vi "Test Event Manager API.vi"() -> ()   [LabVIEW 2022 SP3]
doc: "Event Manager API Tester.\n\n<b>Note:</b> This VI was modified by the <b>Validate DQMH Module</b> tool to add the 'Show Main VI Diagram on Init' functionality included in DQMH 6.1.\n\n<b>Note:</b> This VI was modified by the <b>Validate DQMH Module</b> tool to upgrade its Error Reported event frame to use an improved mechanism for displaying error information.\n\n____\nHAMPEL SOFTWARE ENGINEERING v2.6.0 (2023-12-19 10:54)"
uses:
  Libraries/hse-libraries/Source/hse-dqmh/Controls/Module Display Scenarios.ctl
  <vilib>/Utility/error.llb/DialogType.ctl
  <vilib>/Hampel Software Engineering/HSE Logger/LogRecord/LogRecord.lvclass/LogRecord.ctl
  Event Manager.lvlib
  <vilib>/Hampel Software Engineering/HSE Logger/hse-logger.lvlib
  Libraries/hse-libraries/Source/hse-dqmh/hse-dqmh.lvlib
  <vilib>/Hampel Software Engineering/HSE Logger/LogRecord/LogRecord.lvclass
panel:
  in  "Show Main VI Diagram on Init (F)":bool
  in  "Request UI Display":bool
  in  "Prepare":bool
  in  "Configure":bool
  in  "Scenario":T1
  in  "Set Modules":bool
  in  "Module Paths":path[](array[path])=[path "Modules/Dummie"]
  in  "btn_CRITICAL":bool
  in  "btn_ERROR":bool
  in  "btn_WARNING":bool
  in  "btn_INFO":bool
  in  "btn_DEBUG":bool
  in  "Message":string
  in  "Log Error":errorcluster
  out "Log Record":T2
  in  "Show Block Diagram":bool
  in  "Stop Module":bool
  in  "Start Module":bool
  in  "Hide Module Panel":bool
  in  "Show Module Panel":bool
  out "Status":string
  out "Module Running?":bool
  # "CRITICAL Event"
  # "Generate Event"
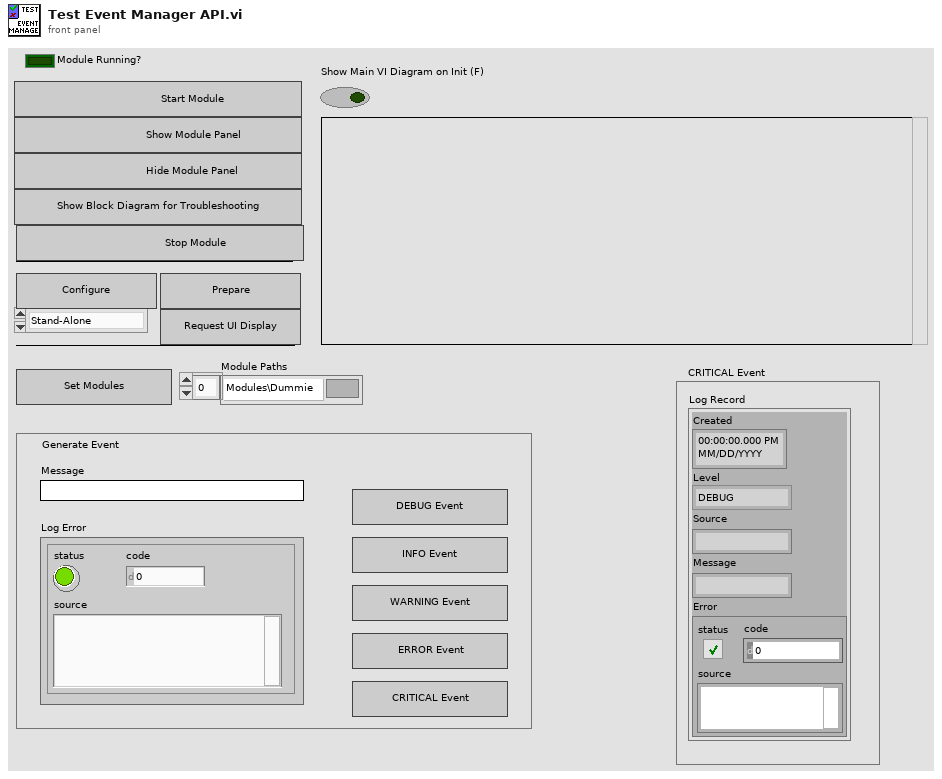
[diagram p1: front panel]
types:
  T1 = typedef "hse-dqmh.lvlib/Module Display Scenarios.ctl" = enum16{"Stand-Alone", "Managed"}
  T2 = cluster{"Created":timestamp, "Level":enum16{"DEBUG", "INFO", "WARNING", "ERROR", "CRITICAL"}, "Source":string, "Message":string, "Error":errorcluster}
  T3 = typedef "Event Manager.lvlib/Broadcast Events--cluster.ctl" = cluster{"Module Did Init":refnum<user-event>, "Status Updated":refnum<user-event>, "Error Reported":refnum<user-event>, "Module Did Stop":refnum<user-event>, "Update Module Execution Status":refnum<user-event>, "System Message":refnum<user-event>}
  T4 = typedef "DialogType.ctl" = u16
  T5 = typedef "hse-dqmh.lvlib/System Message Source.ctl" = enum16{"module", "application", "network"}
  T6 = typedef "hse-logger.lvlib/LogLevel.ctl" = enum16{"DEBUG", "INFO", "WARNING", "ERROR", "CRITICAL"}
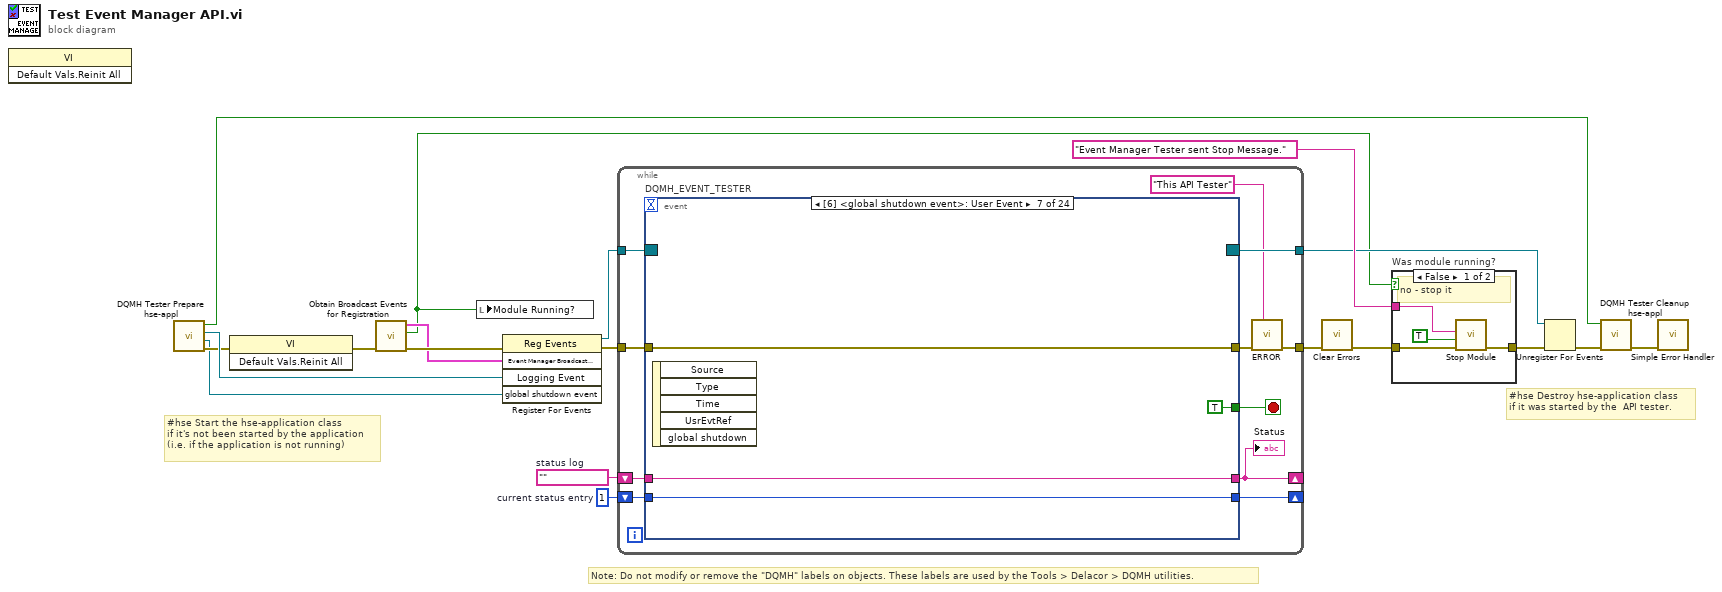
[diagram p0: block diagram]
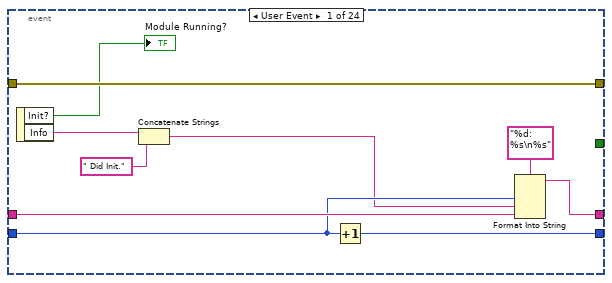
[diagram p3: hidden frame]
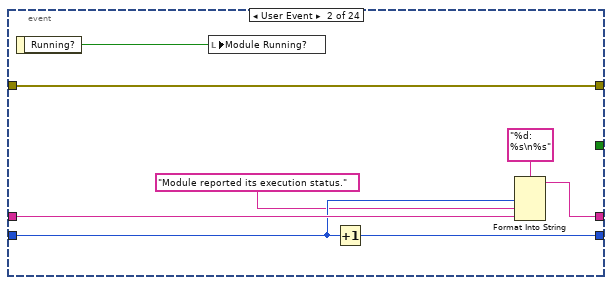
[diagram p4: hidden frame]
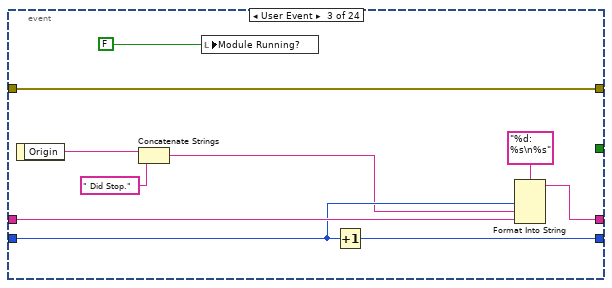
[diagram p5: hidden frame]
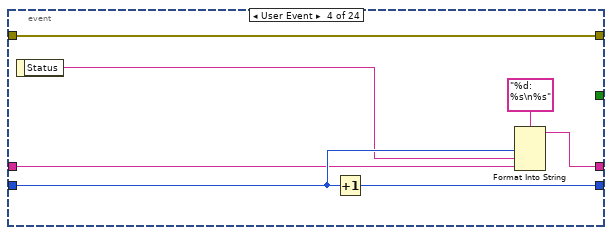
[diagram p6: hidden frame]
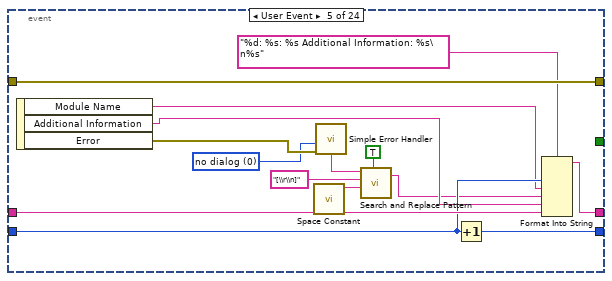
[diagram p7: hidden frame]
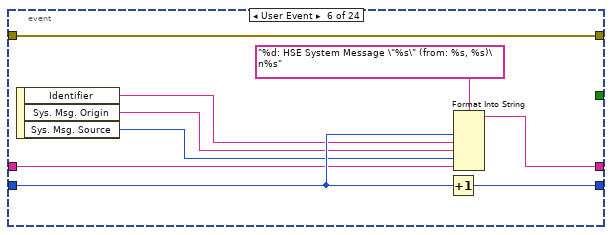
[diagram p8: hidden frame]
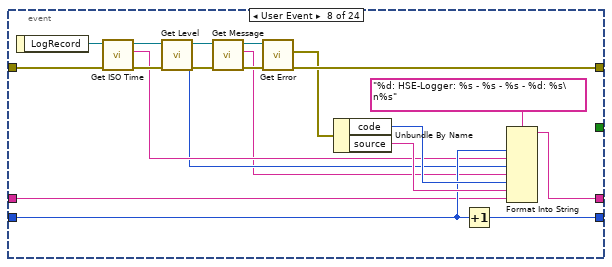
[diagram p9: hidden frame]
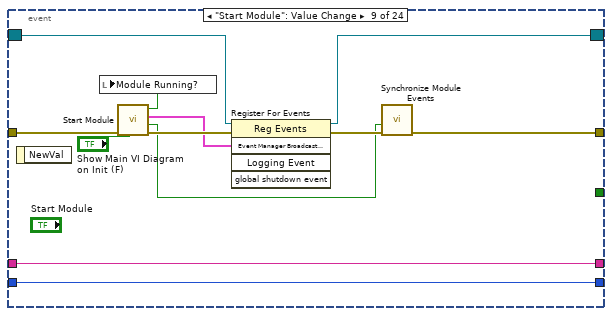
[diagram p10: hidden frame]
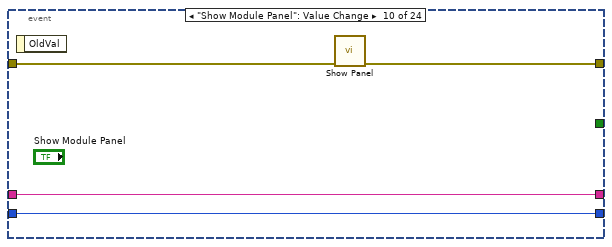
[diagram p11: hidden frame]
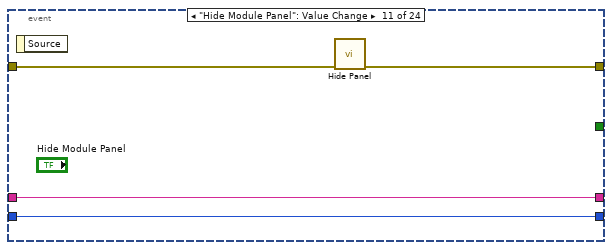
[diagram p12: hidden frame]
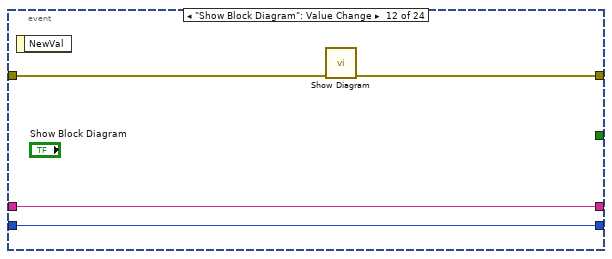
[diagram p13: hidden frame]
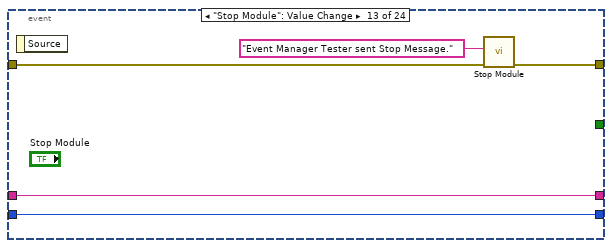
[diagram p14: hidden frame]
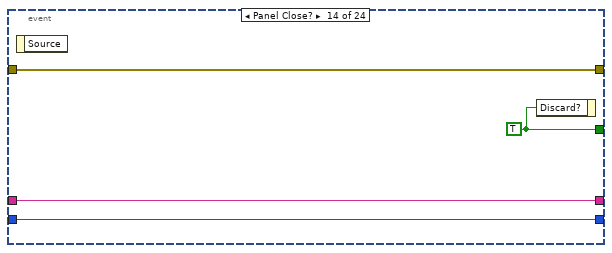
[diagram p15: hidden frame]
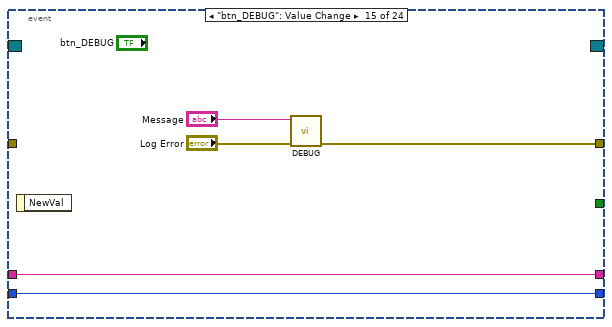
[diagram p16: hidden frame]
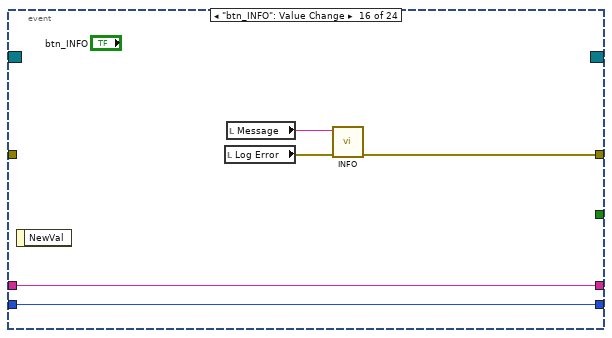
[diagram p17: hidden frame]
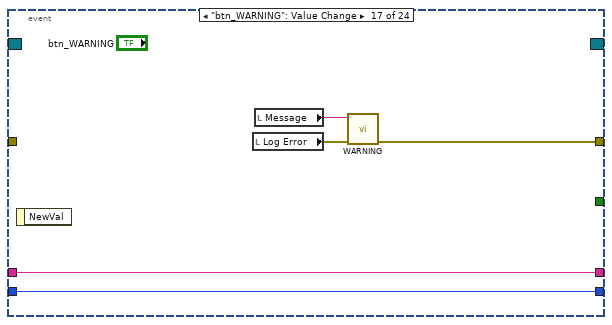
[diagram p18: hidden frame]
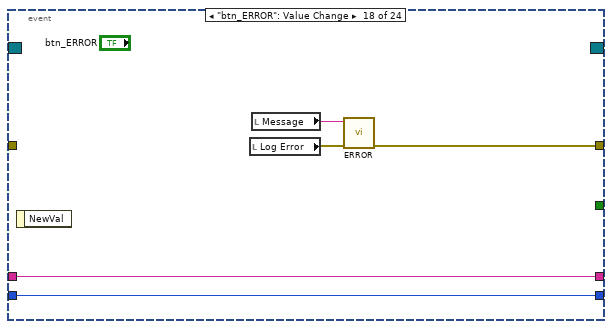
[diagram p19: hidden frame]
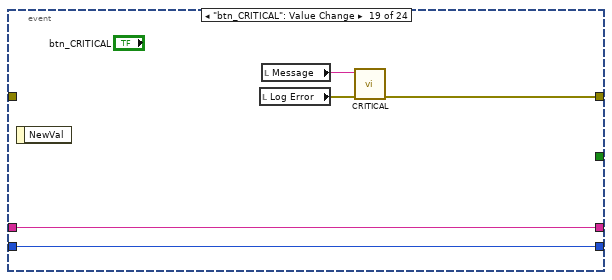
[diagram p20: hidden frame]
diagram:
  w17 = 1  # current status entry
  w18 = ""  # status log
  # "#hse Destroy hse-application class \nif it was started by the  API tester."
  # "#hse Start the hse-application class \nif it's not been started by the application\n(i.e. if the application is not running)"
  # "Note: Do not modify or remove the \"DQMH\" labels on objects. These labels are used by the Tools > Delacor > DQMH utilities."
  n1 = invoke class="VI" method="Default Vals.Reinit All"() -> ()  [unwired: 3 in, 3 out]
  n2 = call "DQMH Tester Prepare hse-appl.vi"() -> ("error out"=w9:errorcluster, "global shutdown event"=w1:refnum<user-event>, "Logging Event"=w10:refnum<user-event>, "Started?"=w12:bool)  [unwired: 8 in]
  n3 = invoke class="VI" method="Default Vals.Reinit All"(error in=w9) -> (error out=w8:errorcluster)  [unwired: 2 in, 2 out]
  n4 = call "Obtain Broadcast Events for Registration.vi"("error in (no error)"=w8) -> ("error out"=w7:errorcluster, "Already running?"=w3:bool, "Event Manager Broadcast Events"=w6:T3)  [unwired: 8 in]
  n5 = local write "Module Running?"(w3) -> ()
  n6 = register-events(error in=w7, w6, w10, w1) -> (reference out=w15:refnum<event-registration>, error out=w16:errorcluster)  [unwired: 1 in]
  n7 = while {
    tunnel: w15 -> [w30]
    tunnel: [w21] -> w13
    shift-right: [w26] -> _
    shift-left: w18 -> [w28]
    shift-right: [w27] -> _
    shift-left: w17 -> [w29]
    tunnel: w16 -> [w25]
    tunnel: [w24] -> w14
    stop <- w22 stop-if-true
    n8 = event "DQMH_EVENT_TESTER" shown="[6] <global shutdown event>: User Event" {
      selector: w30 -> [_ _ _ _ _ _ _ _ w119 _ _ _ _ _ _ _ _ _ _ _ _ _ _ _]
      dyn-events: [_ _ _ _ _ _ _ _ w118 _ _ _ _ _ _ _ _ _ _ _ _ _ _ _] -> w24
      timeout: _ -> [_ _ _ _ _ _ _ _ _ _ _ _ _ _ _ _ _ _ _ _ _ _ _ _]
      tunnel: [_ _ _ _ _ _ TRUE ("Discard?") _ _ _ _ _ _ w146 _ _ _ _ _ _ _ _ _ _] -> w22
      tunnel: [w40 w42 w49 w59 w80 w89 w93 w109 w115 w129 w133 w134 w140 w143 w149 w154 w159 w164 w169 w175 w177 w182 w186 w190] -> w23
      tunnel: w29 -> [w36 w46 w56 w62 w77 w85 w91 w100 w122 w127 w131 w135 w141 w144 w150 w155 w160 w165 w170 w173 w178 w183 w188 w192]
      tunnel: w28 -> [w37 w47 w57 w61 w79 w84 w92 w99 w123 w128 w132 w136 w142 w145 w151 w156 w161 w166 w171 w174 w179 w184 w189 w193]
      tunnel: [w34 w44 w54 w63 w78 w87 w92 w102 w123 w128 w132 w136 w142 w145 w151 w156 w161 w166 w171 w174 w179 w184 w189 w193] -> w26
      tunnel: [w35 w45 w55 w65 w76 w86 w91 w101 w122 w127 w131 w135 w141 w144 w150 w155 w160 w165 w170 w173 w178 w183 w188 w192] -> w27
      tunnel: w25 -> [w40 w42 w49 w59 w80 w89 w93 w110 w117 w126 w130 w137 w138 w143 _ _ _ _ _ w175 w180 w185 w187 w191]
      event User Event {
        n9 = event-data() -> ("Init?"=→"Module Running?":bool, "Info"=w33:string)  [unwired: 1 in]
        n10 = Concatenate Strings(w33, " Did Init.") -> (w32:string)
        n11 = Increment(x=w36) -> (x+1=w35:i32)
        n12 = Format Into String(format string="%d: %s\n%s", w36, w32, w37) -> (resulting string=w34:string)  [unwired: 2 in, 1 out]
      }
      event User Event {
        n13 = event-data() -> ("Running?"=w41:bool)  [unwired: 1 in]
        n14 = local write "Module Running?"(w41) -> ()
        n15 = Increment(x=w46) -> (x+1=w45:i32)
        n16 = Format Into String(format string="%d: %s\n%s", w46, "Module reported its execution status.", w47) -> (resulting string=w44:string)  [unwired: 2 in, 1 out]
      }
      event User Event {
        n17 = event-data() -> ("Origin"=w53:string)  [unwired: 1 in]
        n18 = Concatenate Strings(w53, " Did Stop.") -> (w52:string)
        n19 = local write "Module Running?"(FALSE ("Module Did Init?")) -> ()
        n20 = Increment(x=w56) -> (x+1=w55:i32)
        n21 = Format Into String(format string="%d: %s\n%s", w56, w52, w57) -> (resulting string=w54:string)  [unwired: 2 in, 1 out]
      }
      event User Event {
        n22 = event-data() -> ("Status"=w60:string)  [unwired: 1 in]
        n23 = Increment(x=w62) -> (x+1=w65:i32)
        n24 = Format Into String(format string="%d: %s\n%s", w62, w60, w61) -> (resulting string=w63:string)  [unwired: 2 in, 1 out]
      }
      event User Event {
        w72 = T4 0 items=["no dialog", "OK message", "continue or stop message", "OK message + warnings", "continue/stop + warnings"] ("type of dialog (OK msg:1)")
        n25 = event-data() -> ("Module Name"=w73:string, "Additional Information"=w74:string, "Error"=w75:errorcluster)  [unwired: 1 in]
        n26 = call <vilib>:"Space Constant.vi"() -> ("String"=w68:string)
        n27 = call <vilib>:"Simple Error Handler.vi"("type of dialog (OK msg:1)"=w72, "error in (no error)"=w75) -> ("message"=w71:string)  [unwired: 3 in, 4 out]
        n28 = call <vilib>:"Search and Replace Pattern.vi"("string"=w71, "regular expression (\"\")"="[\\r\\n]" ("regular expression (\"\")"), "replace string (\"\")"=w68, "replace all? (F)"=TRUE ("replace all CR/LF with spaces")) -> ("result string"=w70:string)  [unwired: 1 in, 1 out]
        n29 = Increment(x=w77) -> (x+1=w76:i32)
        n30 = Format Into String(format string="%d: %s: %s Additional Information: %s\n%s", w77, w73, w70, w74, w79) -> (resulting string=w78:string)  [unwired: 2 in, 1 out]
      }
      event User Event {
        n31 = event-data() -> ("Identifier"=w83:string, "Sys. Msg. Origin"=w82:string, "Sys. Msg. Source"=w81:T5)  [unwired: 1 in]
        n32 = Increment(x=w85) -> (x+1=w86:i32)
        n33 = Format Into String(format string="%d: HSE System Message \"%s\" (from: %s, %s)\n%s", w85, w83, w82, w81, w84) -> (resulting string=w87:string)  [unwired: 2 in, 1 out]
      }
      event User Event {
        n34 = event-data() -> ()  [unwired: 1 in, 5 out]
      }
      event User Event {
        n35 = event-data() -> ("LogRecord"=w108:refnum<class "LogRecord.lvclass">)  [unwired: 1 in]
        n36 = call <vilib>:"Get ISO Time.vi"("error in"=w110, "LogRecord in"=w108) -> ("error out"=w113:errorcluster, "ISO Time"=w97:string, "LogRecord out"=w107:refnum<class "LogRecord.lvclass">)  [unwired: 7 in]
        n37 = call <vilib>:"Get Level.vi"("error in"=w113, "LogRecord in"=w107) -> ("error out"=w112:errorcluster, "Level"=w96:T6, "LogRecord out"=w106:refnum<class "LogRecord.lvclass">)  [unwired: 7 in]
        n38 = call <vilib>:"Get Message.vi"("error in"=w112, "LogRecord in"=w106) -> ("error out"=w111:errorcluster, "Message"=w95:string, "LogRecord out"=w105:refnum<class "LogRecord.lvclass">)  [unwired: 7 in]
        n39 = call <vilib>:"Get Error.vi"("error in"=w111, "LogRecord in"=w105) -> ("error out"=w109:errorcluster, "Error"=w98:errorcluster)  [unwired: 7 in, 1 out]
        n40 = Unbundle By Name(w98) -> ("code"=w103:i32, "source"=w104:string)
        n41 = Increment(x=w100) -> (x+1=w101:i32)
        n42 = Format Into String(format string="%d: HSE-Logger: %s - %s - %s - %d: %s\n%s", w100, w97, w96, w95, w103, w104, w99) -> (resulting string=w102:string)  [unwired: 2 in, 1 out]
      }
      event "Start Module": Value Change {
        n43 = event-data() -> ()  [unwired: 1 in, 1 out]
        n44 = call "Start Module.vi"("Show Main VI Diagram on Init (F)"="Show Main VI Diagram on Init (F)", "error in (no error)"=w117) -> ("error out"=w124:errorcluster, "Wait for Event Sync?"=w121:bool, "Event Manager Broadcast Events"=w120:T3, "Module Was Already Running?"=w116:bool)  [unwired: 6 in]
        n45 = local write "Module Running?"(w116) -> ()
        n46 = register-events(reference=w119, error in=w124, w120) -> (reference out=w118:refnum<event-registration>, error out=w125:errorcluster)  [unwired: 2 in]
        n47 = call "Synchronize Module Events.vi"("error in (no error)"=w125, "Wait for Event Sync?"=w121) -> ("error out"=w115:errorcluster)  [unwired: 9 in]
      }
      event "Show Module Panel": Value Change {
        n48 = event-data() -> ()  [unwired: 1 in, 1 out]
        n49 = call "Show Panel.vi"("error in (no error)"=w126) -> ("error out"=w129:errorcluster)  [unwired: 10 in]
      }
      event "Hide Module Panel": Value Change {
        n50 = event-data() -> ()  [unwired: 1 in, 1 out]
        n51 = call "Hide Panel.vi"("error in (no error)"=w130) -> ("error out"=w133:errorcluster)  [unwired: 10 in]
      }
      event "Show Block Diagram": Value Change {
        n52 = event-data() -> ()  [unwired: 1 in, 1 out]
        n53 = call "Show Diagram.vi"("error in (no error)"=w137) -> ("error out"=w134:errorcluster)  [unwired: 10 in]
      }
      event "Stop Module": Value Change {
        n54 = event-data() -> ()  [unwired: 1 in, 1 out]
        n55 = call "Stop Module.vi"("error in (no error)"=w138, "Origin"="Event Manager Tester sent Stop Message.") -> ("error out"=w140:errorcluster)  [unwired: 9 in]
      }
      event Panel Close? {
        w146 = TRUE ("Discard?")
        n56 = event-data() -> ()  [unwired: 1 in, 1 out]
        n57 = event-data("Discard?"=w146) -> ()  [unwired: 1 in, 1 out]
      }
      event "btn_DEBUG": Value Change {
        n58 = event-data() -> ()  [unwired: 1 in, 1 out]
        n59 = call <vilib>:"DEBUG.vi"("Message"="Message", "error in"="Log Error") -> ("error out"=w149:errorcluster)  [unwired: 9 in]
      }
      event "btn_INFO": Value Change {
        n60 = event-data() -> ()  [unwired: 1 in, 1 out]
        n61 = local read "Log Error"() -> (w153:errorcluster)
        n62 = local read "Message"() -> (w152:string)
        n63 = call <vilib>:"INFO.vi"("Message"=w152, "error in"=w153) -> ("error out"=w154:errorcluster)  [unwired: 9 in]
      }
      event "btn_WARNING": Value Change {
        n64 = event-data() -> ()  [unwired: 1 in, 1 out]
        n65 = local read "Log Error"() -> (w158:errorcluster)
        n66 = local read "Message"() -> (w157:string)
        n67 = call <vilib>:"WARNING.vi"("Message"=w157, "error in"=w158) -> ("error out"=w159:errorcluster)  [unwired: 9 in]
      }
      event "btn_ERROR": Value Change {
        n68 = event-data() -> ()  [unwired: 1 in, 1 out]
        n69 = local read "Log Error"() -> (w163:errorcluster)
        n70 = local read "Message"() -> (w162:string)
        n71 = call <vilib>:"ERROR.vi"("Message"=w162, "error in"=w163) -> ("error out"=w164:errorcluster)  [unwired: 9 in]
      }
      event "btn_CRITICAL": Value Change {
        n72 = event-data() -> ()  [unwired: 1 in, 1 out]
        n73 = local read "Log Error"() -> (w168:errorcluster)
        n74 = local read "Message"() -> (w167:string)
        n75 = call <vilib>:"CRITICAL.vi"("Message"=w167, "error in"=w168) -> ("error out"=w169:errorcluster)  [unwired: 9 in]
      }
      event "Log Record": Value Change {
        n76 = event-data() -> ("NewVal"=→"Log Record":T2)  [unwired: 1 in, 1 out]
      }
      event "Set Modules": Value Change {
        n77 = event-data() -> ()  [unwired: 1 in, 6 out]
        n78 = call "Set Modules.vi"("error in (no error)"=w180, "Module Paths"="Module Paths") -> ("error out"=w177:errorcluster)  [unwired: 8 in, 1 out]
      }
      event "Request UI Display": Value Change {
        n79 = event-data() -> ()  [unwired: 1 in, 6 out]
        n80 = call "Request UI Display.vi"("error in (no error)"=w185, "Scenario"="Scenario") -> ("error out"=w182:errorcluster)  [unwired: 8 in, 1 out]
      }
      event "Configure": Value Change {
        n81 = event-data() -> ()  [unwired: 1 in, 6 out]
        n82 = call "Configure.vi"("error in (no error)"=w187) -> ("error out"=w186:errorcluster)  [unwired: 10 in]
      }
      event "Prepare": Value Change {
        n83 = event-data() -> ()  [unwired: 1 in, 6 out]
        n84 = call "Prepare.vi"("error in (no error)"=w191) -> ("error out"=w190:errorcluster)  [unwired: 10 in]
      }
    }
    "Status" <- w26
    n85 = call <vilib>:"ERROR.vi"("Message"="This API Tester" ("Origin"), "error in"=w23) -> ("error out"=w21:errorcluster)  [unwired: 9 in]
  }
  n86 = call <vilib>:"Clear Errors.vi"("error in (no error)"=w13) -> ("error out"=w5:errorcluster)  [unwired: 5 in, 1 out]
  n87 = case "Was module running?" shown="False" w3 {
    tunnel: "Event Manager Tester sent Stop Message." ("Origin") -> [w197 _]
    tunnel: w5 -> [w195 w198]
    tunnel: [w194 w198] -> w4
    frame False {
      # "no - stop it"
      n88 = call "Stop Module.vi"("error in (no error)"=w195, "Wait for Module to Stop? (F)"=TRUE ("Wait for Module to stop?"), "Origin"=w197) -> ("error out"=w194:errorcluster)  [unwired: 8 in]
    }
    frame True {
      # "yes - do nothing"
    }
  }
  n89 = Unregister For Events(event registration refnum=w14, error in=w4) -> (error out=w11:errorcluster)
  n90 = call "DQMH Tester Cleanup hse-appl.vi"("error in"=w11, "Stop?"=w12) -> ("error out"=w2:errorcluster)  [unwired: 9 in]
  n91 = call <vilib>:"Simple Error Handler.vi"("error in (no error)"=w2) -> ()  [unwired: 4 in, 5 out]
